vi "Set Bucket Notification Configuration.vi"(7 "NotificationConfiguration":T1, 8 "error in (no error)":errorcluster, 9 "Bucket":string) -> (0 "error out":errorcluster, 3 "Test message ID":string)   [LabVIEW 2011, in "LV Interface for Amazon S3.lvlib"]
doc: "This operation <B>enables/disables notifications of specified events</B> for a bucket. If the bucket owner and Amazon SNS topic owner are the same, the bucket owner has permission to publish notifications to the topic by default. Otherwise, the owner of the topic must create a policy to enable the bucket owner to publish to the topic. By default, <B>only the bucket owner can configure notifications</B> on a bucket. However, bucket <B>owners can</B> use a bucket policy to <B>grant permission to other users to set this configuration with s3:PutBucketNotification permission</B>. After you call this operation to configure notifications on a bucket, Amazon S3 publishes a test notification to ensure that the topic exists and that the bucket owner has permission to publish to the specified topic. If the notification is successfully published to the SNS topic, the operation updates the bucket configuration and returns the message ID of the test notification sent to topic."
uses:
  LV Interface for Amazon S3.lvlib
  Typedefs/AMZ_S3_API_Setup Bucket Notification Parameters.ctl
  Typedefs/AMZ_S3_Event.ctl
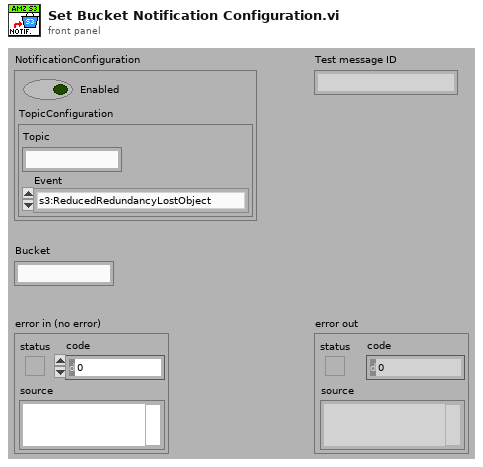
[diagram p1: front panel]
types:
  T1 = typedef "LV Interface for Amazon S3.lvlib/AMZ_S3_API_Setup Bucket Notification Parameters.ctl" = cluster{"Enabled":bool, "TopicConfiguration":cluster{"Topic":string, "Event":T2}}
  T2 = typedef "LV Interface for Amazon S3.lvlib/AMZ_S3_Event.ctl" = enum16{"s3:ReducedRedundancyLostObject"}
  T3 = typedef "LV Interface for Amazon S3.lvlib/AMZ_S3_Call Results.ctl" = enum16{"Success", "UndefinedError", "AccessDenied", "AccountProblem", "AmbiguousGrantByEmailAddress", "BadDigest", "BucketAlreadyExists", "BucketAlreadyOwnedByYou", "BucketNotEmpty", "CredentialsNotSupported", "CrossLocationLoggingProhibited", "EntityTooSmall", "EntityTooLarge", "ExpiredToken", "IllegalVersioningConfigurationException", "IncompleteBody", "IncorrectNumberOfFilesInPostRequest", "InlineDataTooLarge", "InternalError", "InvalidAccessKeyId", "InvalidAddressingHeader", "InvalidArgument", "InvalidBucketName", "InvalidDigest", "InvalidLocationConstraint", "InvalidPart", "InvalidPartOrder", "InvalidPayer", "InvalidPolicyDocument", "InvalidRange", "InvalidSecurity", "InvalidSOAPRequest", "InvalidStorageClass", "InvalidTargetBucketForLogging", "InvalidToken", "InvalidURI", "KeyTooLong", "MalformedACLError", "MalformedPOSTRequest", "MalformedXML", "MaxMessageLengthExceeded", "MaxPostPreDataLengthExceededError", "MetadataTooLarge", "MethodNotAllowed", "MissingAttachment", "MissingContentLength", "MissingRequestBodyError", "MissingSecurityElement", "MissingSecurityHeader", "NoLoggingStatusForKey", "NoSuchBucket", "NoSuchKey", "NoSuchUpload", "NoSuchVersion", "NotImplemented", "NotSignedUp", "OperationAborted", "PermanentRedirect", "PreconditionFailed", "Redirect", "RequestIsNotMultiPartContent", "RequestTimeout", "RequestTimeTooSkewed", "RequestTorrentOfBucketError", "SignatureDoesNotMatch", "SlowDown", "TemporaryRedirect", "TokenRefreshRequired", "TooManyBuckets", "UnexpectedContent", "UnresolvableGrantByEmailAddress", "UserKeyMustBeSpecified", "LabVIEWError"}
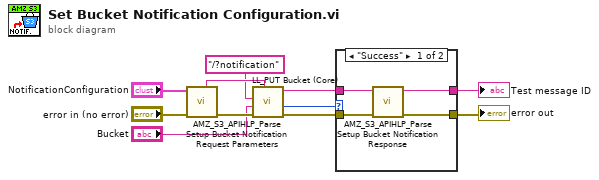
[diagram p0: block diagram]
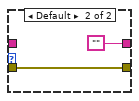
[diagram p2: hidden frame]
diagram:
  n1 = call "AMZ_S3_APIHLP_Parse Setup Bucket Notification Request Parameters.vi"("error in (no error)"="error in (no error)", "Setup Notification Request parameters"="NotificationConfiguration") -> ("error out"=w9:errorcluster, "PUT Data"=w8:string)  [unwired: 8 in]
  n2 = call "LL_PUT Bucket (Core).vi"("Data"=w8, "error in (no error)"=w9, "Bucket"="Bucket", "Path and query string"="/?notification") -> ("error out"=w4:errorcluster, "Call Result"=w5:T3, "Response header"=w3:string)  [unwired: 4 in, 1 out]
  n3 = case shown="\"Success\"" w5 {
    tunnel: w4 -> [w15 w17]
    tunnel: w3 -> [w14 _]
    tunnel: [w13 ""] -> w1
    tunnel: [w12 w17] -> w2
    frame "Success" {
      n4 = call "AMZ_S3_APIHLP_Parse Setup Bucket Notification Response.vi"("error in (no error)"=w15, "Response header"=w14) -> ("error out"=w12:errorcluster, "Test message id"=w13:string)  [unwired: 8 in]
    }
    frame Default {
    }
  }
  "Test message ID" <- w1
  "error out" <- w2
